vi "Tester.vi"   [LabVIEW 2012, in "Architecture.lvlib"]
uses:
  Architecture.lvlib
  Thread/Thread.lvclass
  Queue/Queue.lvclass
  Message/Message.lvclass
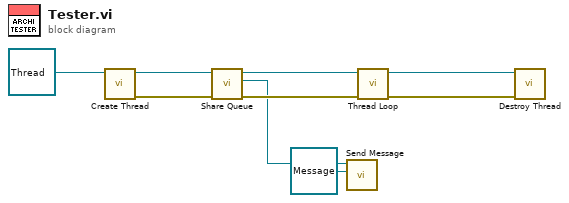
[diagram p0: block diagram]
diagram:
  n1 = call-dynamic "Create Thread.vi"("Thread in"=refnum<class "Thread.lvclass"> refnum) -> ("error out"=w6:errorcluster, "Thread out"=w8:refnum<class "Thread.lvclass">)  [unwired: 9 in]
  n2 = call "Share Queue.vi"("error in (no error)"=w6, "Thread in"=w8) -> ("error out"=w5:errorcluster, "Architecture.lvlib:Queue.lvclass"=w4:refnum<class "Queue.lvclass">, "Thread out"=w7:refnum<class "Thread.lvclass">)  [unwired: 7 in]
  n3 = call "Send Message.vi"("Architecture.lvlib:Message.lvclass"=refnum<class "Message.lvclass"> refnum, "Queue in"=w4) -> ()  [unwired: 8 in, 2 out]
  n4 = call-dynamic "Thread Loop.vi"("error in (no error)"=w5, "Thread in"=w7) -> ("error out"=w1:errorcluster, "Thread out"=w2:refnum<class "Thread.lvclass">)  [unwired: 8 in]
  n5 = call-dynamic "Destroy Thread.vi"("error in (no error)"=w1, "Thread in"=w2) -> ()  [unwired: 9 in, 1 out]
